vi "VISA Command.vi"(8 "error in":errorcluster, 10 "Command":string, 11 "VISA name in":refnum<visa-resource-name>) -> (0 "error out":errorcluster, 2 "Return":string, 3 "VISA name out":refnum<visa-resource-name>)   [LabVIEW 2019, in "Allmotion.lvlib"]
uses:
  Allmotion.lvlib
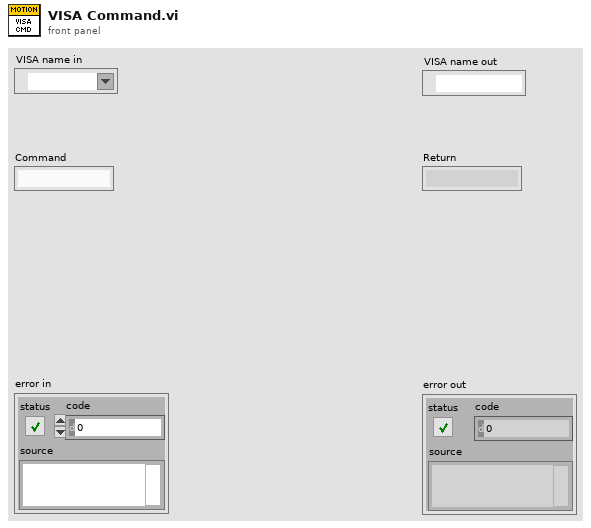
[diagram p1: front panel]
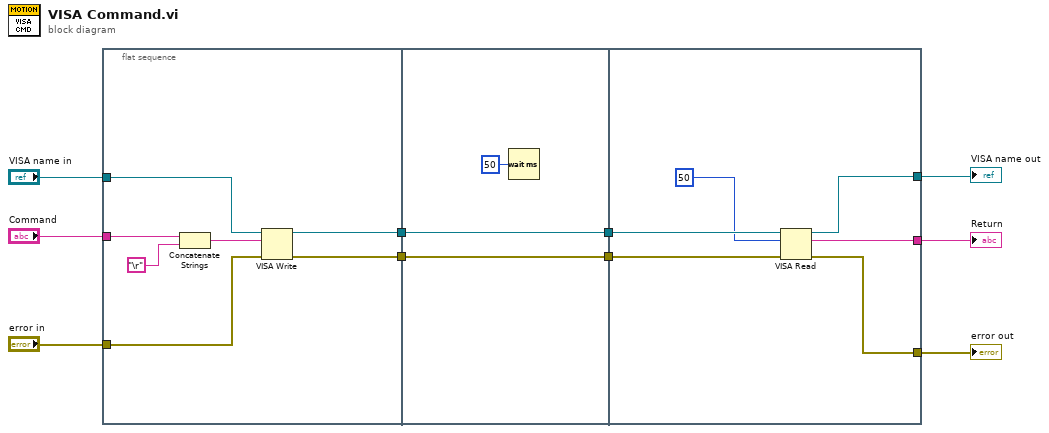
[diagram p0: block diagram]
diagram:
  n1 = flat-sequence {
    tunnel: "Command" -> [w17]
    tunnel: "VISA name in" -> [w14]
    tunnel: "error in" -> [w13]
    tunnel: [w12] -> w6
    tunnel: [w11] -> w4
    tunnel: [w19] -> w7
    tunnel: w6 -> [w19]
    tunnel: [w18] -> w5
    tunnel: w4 -> [w18]
    tunnel: w7 -> [w26]
    tunnel: w5 -> [w25]
    tunnel: [w23] -> w2
    tunnel: [w22] -> w3
    tunnel: [w21] -> w1
    frame #0 {
      n2 = Concatenate Strings(w17, "\r") -> (w15:string)
      n3 = VISA Write(VISA resource name=w14, write buffer=w15, error in (no error)=w13) -> (VISA resource name out=w12:refnum<visa-resource-name>, error out=w11:errorcluster)  [unwired: 1 out]
    }
    frame #1 {
      n4 = Wait (ms)(milliseconds to wait=u32 50) -> ()  [unwired: 1 out]
    }
    frame #2 {
      n5 = VISA Read(VISA resource name=w26, byte count=u32 50, error in (no error)=w25) -> (VISA resource name out=w23:refnum<visa-resource-name>, read buffer=w21:string, error out=w22:errorcluster)  [unwired: 1 out]
    }
  }
  "error out" <- w3
  "VISA name out" <- w2
  "Return" <- w1
